vi "WriteBin.vi"(8 "error in (no error)":errorcluster, 9 "operation (0:open)":T1(ring), 10 "BinaryEncoding":u8[](array[numeric]), 11 "appended path":path) -> (0 "error out":errorcluster, 3 "path":path)   [LabVIEW 2020]
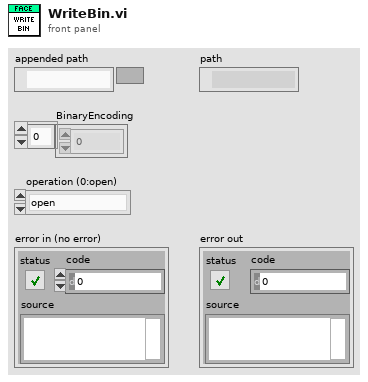
[diagram p1: front panel]
types:
  T1 = enum16{"open", "replace", "create", "open or create", "replace or create", "replace or create with confirmation"}
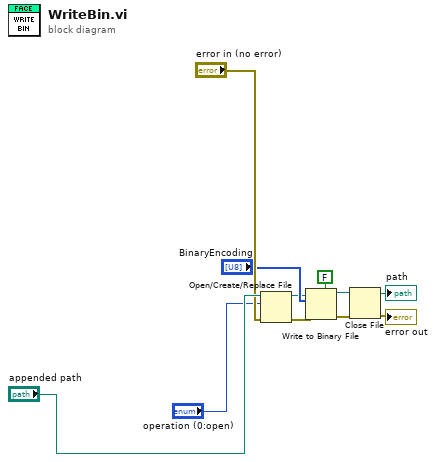
[diagram p0: block diagram]
diagram:
  n1 = Open/Create/Replace File(file path (use dialog)="appended path", error in="error in (no error)", operation (0:open)="operation (0:open)") -> (refnum out=w5:refnum<file>, error out=w1:errorcluster)  [unwired: 3 in, 1 out]
  n2 = Write to Binary File(file (use dialog)=w5, data="BinaryEncoding", error in=w1, 5:FALSE ("prepend array or string size? (T)")) -> (refnum out=w3:refnum<file>, error out=w2:errorcluster)  [unwired: 2 in, 1 out]
  n3 = Close File(refnum=w3, error in=w2) -> (path=→"path":path, error out=→"error out":errorcluster)
